vi "NF87XX.set i Attr.vi"(2 "error in (no error)":errorcluster, 3 "DB Entry to read":string) -> (0 "error out":errorcluster, 1 "i Attributes":T1={"Con Settings"={"VISA or TCP/IP"=FALSE, "Init Connection"=TRUE, "Close Connection"=FALSE, "Resource Name"="COM1", "hostname"="N/A", "connection ID"=refnum}, "Drivers"=[], "Status"={"Service ID"=-1, "Status"=0}, "Joystick available"=FALSE, "VISA Resource"="N/A"} {"Status"."Status" items=["no info", "off/false/out", "on/true/in", "Failure", "Alarm", "Status 1", "Status 2", "Status 3"]})   [LabVIEW 2014, in "NF87XX.lvlib"]
uses:
  NF87XX.lvlib
  NF87XX.i attribute.ctl
  non_GPL/instr.lib/NewFocusPico/VISA & TCPIP Control.ctl
  NF87XX.driver Settings.ctl
  NF87XX.driver Type.ctl
  non_GPL/instr.lib/NewFocusPico/Pico Parameters.ctl
  CSPhelix/PH_StatusHandler/PH_StatusHandler.Status.ctl
  CSPhelix/PH_Common/PH_Common.lvlib
  non_GPL/instr.lib/NewFocusPico/NewFocusPico - Driver np.lvlib
  CSPhelix/PH_StatusHandler/PH_StatusHandler.lvlib
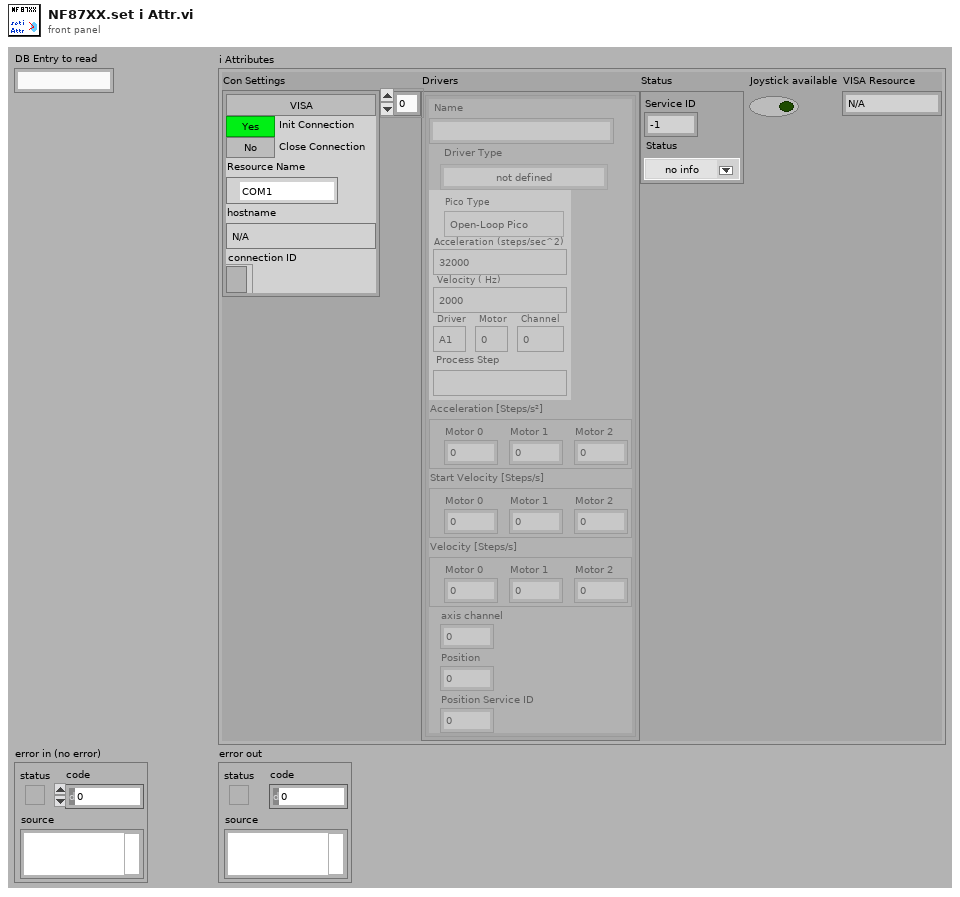
[diagram p1: front panel]
types:
  T1 = typedef "NF87XX.lvlib/NF87XX.i attribute.ctl" = cluster{"Con Settings":T2, "Drivers":T3[], "Status":cluster{"Service ID":i32, "Status":T6}, "Joystick available":bool, "VISA Resource":string}
  T2 = typedef "NewFocusPico - Driver np.lvlib/VISA & TCPIP Control.ctl" = cluster{"VISA or TCP/IP":bool, "Init Connection":bool, "Close Connection":bool, "Resource Name":refnum<visa-resource-name>, "hostname":string, "connection ID":refnum<k5>}
  T3 = typedef "NF87XX.lvlib/NF87XX.driver Settings.ctl" = cluster{"Name":string, "Driver Type":T4, "Pico Parameter type":T5, "Acceleration [Steps/s²]":cluster{"Motor 0":dbl, "Motor 1":dbl, "Motor 2":dbl}, "Start Velocity [Steps/s]":cluster{"Motor 0":dbl, "Motor 1":dbl, "Motor 2":dbl}, "Velocity [Steps/s]":cluster{"Motor 0":dbl, "Motor 1":dbl, "Motor 2":dbl}, "axis channel":i32, "Position":i32, "Position Service ID":i32}
  T4 = typedef "NF87XX.lvlib/NF87XX.driver Type.ctl" = enum16{"not defined", "3-ch open loop drv", "1-ch closed loop drv"}
  T5 = typedef "NewFocusPico - Driver np.lvlib/Pico Parameters.ctl" = cluster{"Pico Type":enum16{"Open-Loop Pico", "Close-Loop Pico", "Pico Ultra"}, "Acceleration (steps/sec^2)":string, "Velocity ( Hz)":string, "Driver":string, "Motor":string, "Channel":string, "Process Step":string}
  T6 = typedef "PH_StatusHandler.lvlib/PH_StatusHandler.Status.ctl" = i16
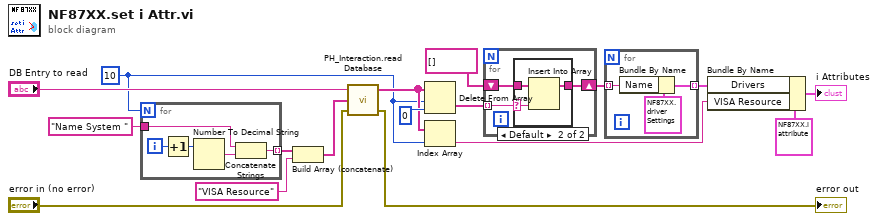
[diagram p0: block diagram]
diagram:
  w1 = 10
  n1 = for {
    N: w1 -> [_]
    tunnel: "Name System " -> [w19]
    tunnel: [w18] -> w13 mode=indexing
    i -> [w22]
    n2 = Increment(x=w22) -> (x+1=w21:i32)
    n3 = Number To Decimal String(number=w21) -> (decimal integer string=w20:string)  [unwired: 1 in]
    n4 = Concatenate Strings(w19, w20) -> (w18:string)
  }
  n5 = Build Array (concatenate)(w13, "VISA Resource") -> (w11:string[])
  n6 = call "PH_Interaction.read Database.vi"("error in (no error)"="error in (no error)", "Strings to search for"=w11, "DB Entry to read"="DB Entry to read") -> ("error out"=→"error out":errorcluster, "Values"=w8:string[])  [unwired: 1 in]
  n7 = Delete From Array(array=w8, length=w1, index=0) -> (deleted portion=w9:string[])  [unwired: 1 out]
  n8 = Index Array(array=w8, index=w1) -> (element=w7:string)
  n9 = for {
    tunnel: w9 -> [w23] mode=indexing
    shift-right: [w24] -> w16
    shift-left: string[] [] -> [w25]
    n10 = case shown="Default" w23 {
      selector: w23 -> [_ w27]
      tunnel: w25 -> [w26 w29]
      tunnel: [w26 w28] -> w24
      frame "", "N/A" {
      }
      frame Default {
        n11 = Insert Into Array(array=w29, new element=w27) -> (w28:string[])  [unwired: 1 in]
      }
    }
  }
  n12 = for {
    tunnel: w16 -> [w32] mode=indexing
    tunnel: [w31] -> w6 mode=indexing
    n13 = Bundle By Name(cluster=T3 {"Name"="", "Driver Type"=enum."not defined", "Pico Parameter type"={"Pico Type"=enum."Open-Loop Pico", "Acceleration (steps/sec^2)"="32000", "Velocity ( Hz)"="2000", "Driver"="A1", "Motor"="0", "Channel"="0", "Process Step"=""}, "Acceleration [Steps/s²]"={"Motor 0"=0.0, "Motor 1"=0.0, "Motor 2"=0.0}, "Start Velocity [Steps/s]"={"Motor 0"=0.0, "Motor 1"=0.0, "Motor 2"=0.0}, "Velocity [Steps/s]"={"Motor 0"=0.0, "Motor 1"=0.0, "Motor 2"=0.0}, "axis channel"=0, "Position"=0, "Position Service ID"=0} ("element"), "Name"=w32) -> (w31:T3)
  }
  n14 = Bundle By Name(cluster=T1 {"Con Settings"={"VISA or TCP/IP"=FALSE, "Init Connection"=TRUE, "Close Connection"=FALSE, "Resource Name"="COM1", "hostname"="N/A", "connection ID"=refnum}, "Drivers"=[], "Status"={"Service ID"=-1, "Status"=0}, "Joystick available"=FALSE, "VISA Resource"="N/A"} ("i Attributes 2"), "Drivers"=w6, "VISA Resource"=w7) -> (→"i Attributes":T1)
